vi "Read Sample Rate.vi"(8 "error in (no error)":errorcluster, 11 "PXIe5105 in":refnum<class "PXIe5105.lvclass">) -> (0 "error out":errorcluster, 2 "Sample Rate":dbl, 3 "PXIe5105 out":refnum<class "PXIe5105.lvclass">)   [LabVIEW 2018, in "PXIe5105.lvlib" / "PXIe5105.lvclass"]
uses:
  PXIe5105.lvclass
  PXIe5105.lvclass/PXIe5105.ctl
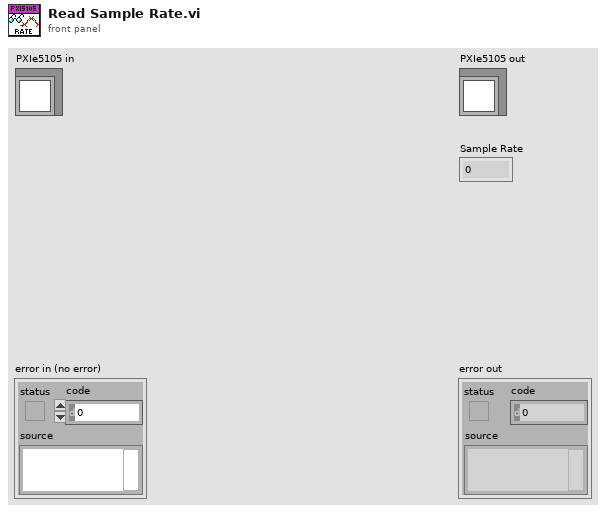
[diagram p1: front panel]
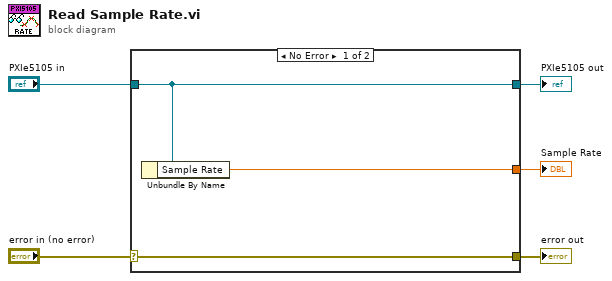
[diagram p0: block diagram]
diagram:
  n1 = case shown="No Error" "error in (no error)" {
    selector: "error in (no error)" -> [w8 w9]
    tunnel: [w8 w9] -> w4
    tunnel: [w7 w10] -> w2
    tunnel: "PXIe5105 in" -> [w7 w10]
    tunnel: [w6 _] -> w1
    frame No Error {
      n2 = Unbundle By Name(w7) -> ("Sample Rate"=w6:dbl)
    }
    frame Error {
    }
  }
  "error out" <- w4
  "PXIe5105 out" <- w2
  "Sample Rate" <- w1
